vi "Correct.vi"(10 "Input":variant, 11 "Data in":waveform(dbl)[](array[waveform])) -> (1 "Incorrect movement":bool, 2 "Correct movement":bool, 3 "Centered":bool)   [LabVIEW 2011]
uses:
  Z:/libraries/Labview/Trial Based Experiment/TYPE - State triggers.ctl
  <vilib>/Analysis/NI_AALBase.lvlib
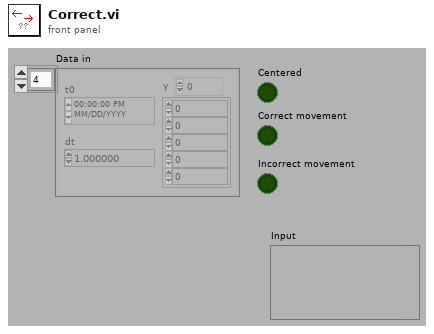
[diagram p1: front panel]
types:
  T1 = typedef "TYPE - State triggers.ctl" = enum16{"Start Session", "Start Trial", "Intertrial", "Acquire Fixation", "Delay Period", "Response Period", "Reward", "Abort Trial", "End Trial"}
  T2 = cluster{"Trial Type":i32, "Joystick Threshold":dbl, "Fixation Radius":dbl, "Left Target":dbl[][], "Right Target":dbl[][], "Target Radius":dbl, "Trigger":T1}
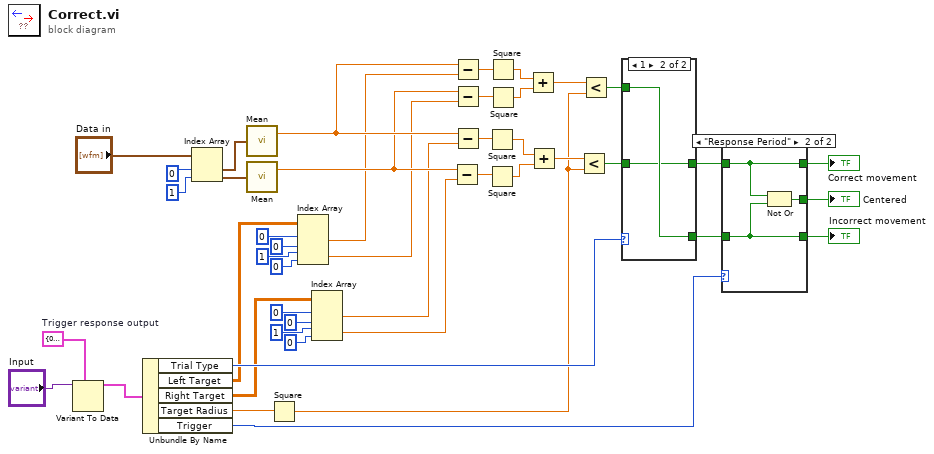
[diagram p0: block diagram]
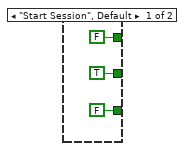
[diagram p2: hidden frame]
diagram:
  w12 = T2 {"Trial Type"=0, "Joystick Threshold"=0.0, "Fixation Radius"=0.0, "Left Target"=[], "Right Target"=[], "Target Radius"=0.0, "Trigger"=enum."End Trial"}  # Trigger response output
  n1 = Variant To Data(type=w12, Variant="Input") -> (data=w38:T2)  [unwired: 1 in, 1 out]
  n2 = Unbundle By Name(w38) -> ("Trial Type"=w39:i32, "Left Target"=w35:dbl[][], "Right Target"=w28:dbl[][], "Target Radius"=w17:dbl, "Trigger"=w6:T1)
  n3 = Index Array(array="Data in", index #1=0 ("index"), index #2=1 ("index")) -> (element #1=w42:waveform(dbl), element #2=w41:waveform(dbl))
  n4 = call <vilib>:"Mean.vi"("X"=w42) -> ("mean"=w27:dbl)  [unwired: 1 out]
  n5 = call <vilib>:"Mean.vi"("X"=w41) -> ("mean"=w26:dbl)  [unwired: 1 out]
  n6 = Square(x=w17) -> (x^2=w7:dbl)
  n7 = Index Array(array=w35, index (row) #1=0 ("index"), index (col) #1=0 ("disabled index (col)"), index (row) #2=1 ("index"), index (col) #2=0 ("disabled index (col)")) -> (element #1=w11:dbl, element #2=w10:dbl)
  n8 = Index Array(array=w28, index (row) #1=0 ("index"), index (col) #1=0 ("disabled index (col)"), index (row) #2=1 ("index"), index (col) #2=0 ("disabled index (col)")) -> (element #1=w9:dbl, element #2=w8:dbl)
  n9 = Subtract(x=w26, y=w8) -> (x-y=w25:dbl)
  n10 = Subtract(x=w27, y=w11) -> (x-y=w24:dbl)
  n11 = Subtract(x=w26, y=w10) -> (x-y=w23:dbl)
  n12 = Subtract(x=w27, y=w9) -> (x-y=w22:dbl)
  n13 = Square(x=w22) -> (x^2=w18:dbl)
  n14 = Square(x=w25) -> (x^2=w19:dbl)
  n15 = Square(x=w24) -> (x^2=w20:dbl)
  n16 = Square(x=w23) -> (x^2=w21:dbl)
  n17 = Add(x=w20, y=w21) -> (x+y=w15:dbl)
  n18 = Add(x=w18, y=w19) -> (x+y=w16:dbl)
  n19 = Less?(x=w16, y=w7) -> (x < y?=w13:bool)
  n20 = Less?(x=w15, y=w7) -> (x < y?=w14:bool)
  n21 = case shown="1" w39 {
    tunnel: [w47 w48] -> w4
    tunnel: w14 -> [w47 w49]
    tunnel: [w46 w49] -> w3
    tunnel: w13 -> [w46 w48]
    frame 0, Default {
    }
    frame 1 {
    }
  }
  n22 = case shown="\"Response Period\"" w6 {
    tunnel: [TRUE w55] -> w5
    tunnel: w4 -> [_ w54]
    tunnel: w3 -> [_ w53]
    tunnel: [FALSE w54] -> w2
    tunnel: [FALSE w53] -> w1
    frame "Start Session", Default {
    }
    frame "Response Period" {
      n23 = Not Or(1:w53, 2:w54) -> (0:w55:bool)
    }
  }
  "Centered" <- w5
  "Correct movement" <- w2
  "Incorrect movement" <- w1
